vi "LINC Close.vi"(8 "error in (no error)":errorcluster, 11 "LINC session":refnum<class "LINC.lvclass">) -> (0 "error out":errorcluster)   [LabVIEW 2018, in "STEPkgDriver_LINC.lvlib" / "LINC.lvclass"]
uses:
  LINC.lvclass
  STEPkgDriver_LINC.lvlib
  LINC Global Mode.ctl
  LINC Global Config Mode.ctl
  LINC Global Session Mode.ctl
  LINC Global Handshake Mode.ctl
  LINC Global ID Mode.ctl
  LINC Daemon Manager Mode.ctl
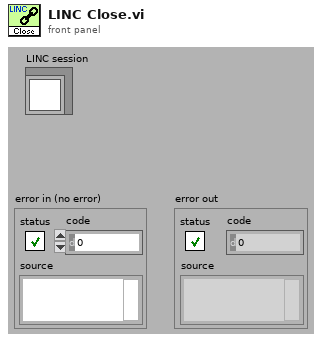
[diagram p1: front panel]
types:
  T1 = typedef "STEPkgDriver_LINC.lvlib/LINC Daemon Manager Mode.ctl" = enum16{"INIT", "CLEAR", "GET"}
  T2 = typedef "STEPkgDriver_LINC.lvlib/LINC Global ID Mode.ctl" = enum16{"INIT", "CLEAR", "GET_ID"}
  T3 = typedef "STEPkgDriver_LINC.lvlib/LINC Global Handshake Mode.ctl" = enum16{"INIT", "CLEAR", "ADD_COMMAND", "RMV_COMMAND", "CLR_HANDSHAKE", "SET_HANDSHAKE", "GET_HANDSHAKE"}
  T4 = typedef "STEPkgDriver_LINC.lvlib/LINC Global Session Mode.ctl" = enum16{"INIT", "CLEAR", "ADD_SESSION", "SET_CONNECTION", "SET_LISTENER", "SET_REFERENCE", "GET_SESSION"}
  T5 = typedef "STEPkgDriver_LINC.lvlib/LINC Global Config Mode.ctl" = enum16{"INIT", "CLEAR", "SET_CMD_CB", "SET_TLM_CB", "SET_CMD_FIELDS", "SET_TLM_FIELDS", "SET_ID", "GET_CONFIG"}
  T6 = typedef "STEPkgDriver_LINC.lvlib/LINC Global Mode.ctl" = enum16{"INIT", "CLEAR", "ADD_PKT_HDR", "ADD_PKT", "GET_PKT_NAMES", "GET_PKT_DESC", "GET_PKT_HDR", "GET_PKT", "SET_PKT", "SET_DATA", "SIM_EN", "SIM_DS"}
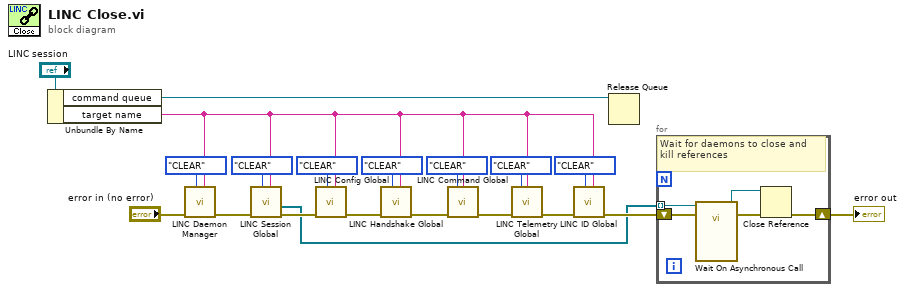
[diagram p0: block diagram]
diagram:
  n1 = Unbundle By Name("LINC session") -> ("command queue"=w13:refnum<queue>, "target name"=w5:string)
  n2 = call "LINC Daemon Manager.vi"("target name"=w5, "mode"=LINC_Daemon_Manager_Mode."CLEAR", "error in (no error)"="error in (no error)") -> ("error out"=w6:errorcluster)  [unwired: 7 in, 1 out]
  n3 = call "LINC Session Global.vi"("target name"=w5, "mode"=LINC_Global_Session_Mode."CLEAR", "error in (no error)"=w6) -> ("error out"=w15:errorcluster, "reference out"=w1:refnum<vi>[])  [unwired: 4 in, 3 out]
  n4 = call "LINC Config Global.vi"("target name"=w5, "mode"=LINC_Global_Config_Mode."CLEAR", "error in (no error)"=w15) -> ("error out"=w12:errorcluster)  [unwired: 7 in, 1 out]
  n5 = call "LINC Handshake Global.vi"("target name"=w5, "mode"=LINC_Global_Handshake_Mode."CLEAR", "error in (no error)"=w12) -> ("error out"=w11:errorcluster)  [unwired: 5 in, 3 out]
  n6 = call "LINC Command Global.vi"("mode"=LINC_Global_Mode."CLEAR", "target name"=w5, "error in (no error)"=w11) -> ("error out"=w20:errorcluster)  [unwired: 8 in, 4 out]
  n7 = call "LINC Telemetry Global.vi"("mode"=LINC_Global_Mode."CLEAR", "target name"=w5, "error in (no error)"=w20) -> ("error out"=w9:errorcluster)  [unwired: 8 in, 4 out]
  n8 = call "LINC ID Global.vi"("target name"=w5, "mode"=LINC_Global_ID_Mode."CLEAR", "error in (no error)"=w9) -> ("error out"=w3:errorcluster)  [unwired: 7 in, 1 out]
  n9 = Release Queue(queue=w13) -> ()  [unwired: 2 in, 3 out]
  n10 = for {
    shift-right: [w22] -> w2
    shift-left: w3 -> [w23]
    tunnel: w1 -> [w21] mode=indexing
    # "Wait for daemons to close and kill references"
    n11 = call-by-ref "Wait On Asynchronous Call"(reference=w21, error in=w23) -> (reference out=w24:refnum<vi>, error out=w25:errorcluster)  [unwired: 12 in]
    n12 = Close Reference(reference=w24, error in (no error)=w25) -> (error out=w22:errorcluster)
  }
  "error out" <- w2
